vi "FPGA Encode.vi"(7 "Reset ENC":bool, 10 "B":bool, 11 "A":bool) -> (3 "ENC":i32)   [LabVIEW 2017]
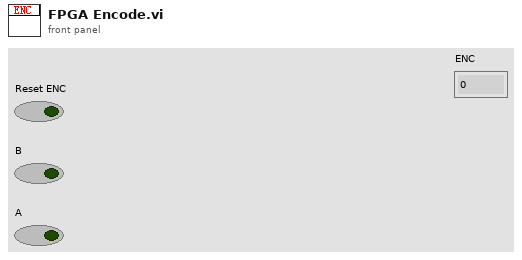
[diagram p1: front panel]
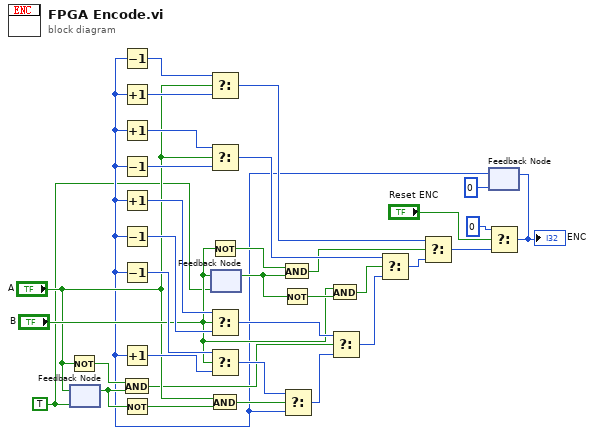
[diagram p0: block diagram]
diagram:
  w1 = TRUE ("B")
  n1 = Not(x="A") -> (.not. x?=w28:bool)
  n2 = feedback #1(w1) -> (w8:bool)
  n3 = feedback-in #1("A") -> ()
  n4 = And(x=w28, y=w8) -> (x .and. y?=w7:bool)
  n5 = Not(x=w8) -> (.not. x?=w29:bool)
  n6 = Not(x="B") -> (.not. x?=w21:bool)
  n7 = And(x="A", y=w29) -> (x .and. y?=w27:bool)
  n8 = feedback #2(w1) -> (w9:bool)
  n9 = feedback-in #2("B") -> ()
  n10 = And(x=w21, y=w9) -> (x .and. y?=w11:bool)
  n11 = Not(x=w9) -> (.not. x?=w20:bool)
  n12 = And(x="B", y=w20) -> (x .and. y?=w16:bool)
  n13 = feedback #3(0) -> (w2:i32)
  n14 = Decrement(x=w2) -> (x-1=w33:i32)
  n15 = Increment(x=w2) -> (x+1=w34:i32)
  n16 = Increment(x=w2) -> (x+1=w14:i32)
  n17 = Decrement(x=w2) -> (x-1=w15:i32)
  n18 = Increment(x=w2) -> (x+1=w24:i32)
  n19 = Decrement(x=w2) -> (x-1=w25:i32)
  n20 = Decrement(x=w2) -> (x-1=w31:i32)
  n21 = Increment(x=w2) -> (x+1=w30:i32)
  n22 = Select(t=w33, s="A", f=w34) -> (s? t:f=w13:i32)
  n23 = Select(t=w14, s="A", f=w15) -> (s? t:f=w12:i32)
  n24 = Select(t=w24, s="B", f=w25) -> (s? t:f=w23:i32)
  n25 = Select(t=w31, s="B", f=w30) -> (s? t:f=w26:i32)
  n26 = Select(t=w26, s=w27, f=w2) -> (s? t:f=w22:i32)
  n27 = Select(t=w23, s=w7, f=w22) -> (s? t:f=w18:i32)
  n28 = Select(t=w12, s=w16, f=w18) -> (s? t:f=w17:i32)
  n29 = Select(t=w13, s=w11, f=w17) -> (s? t:f=w6:i32)
  n30 = Select(t=0, s="Reset ENC", f=w6) -> (s? t:f=w3:i32)
  "ENC" <- w3
  n31 = feedback-in #3(w3) -> ()
